vi "Test Dataset.vi"(11 "Enum":T1(ring)) -> (0 "error out":errorcluster, 2 "Parameters out":dbl[](array[numeric])=[-9.0, -8.75, -8.5, -8.25, -8.0, -7.75, -7.5, -7.25, -7.0, -6.75, -6.5, -6.25, -6.0, -5.75, -5.5, -5.25, -5.0, -4.75, -4.5, -4.25, -4.0, -3.75, -3.5, -3.25, -3.0, -2.75, -2.5, -2.25, -2.0, -1.75, -1.5, -1.25, -1.0, -0.75, -0.5, -0.25, 0.0, 0.25, 0.5, 0.75, 1.0, 1.25, 1.5, 1.75, 2.0, 2.25, 2.5, 2.75, 3.0, 3.25, 3.5, 3.75, 4.0, 4.25, 4.5, 4.75, 5.0, 5.25, 5.5, 5.75, 6.0, 6.25, 6.5, 6.75, 7.0, 7.25, 7.5, 7.75, 8.0, 8.25, 8.5, 8.75, 9.0], 3 "XY-data out":cluster{"X-array":dbl[], "Y-array":dbl[]}[](array[cluster]) {"Y-array" format="%.2p"; "X-array" format="%.2p"})   [LabVIEW 2019, in "xy_utilities.lvlib"]
uses:
  <vilib>/Utility/miscctls.llb/LVOffsetAndMultiplierTypeDef.ctl
  subVIs/Append (multiple).vi
  subVIs/Subtract float (multiple).vi
  subVIs/Append (single).vi
  subVIs/Append (double array).vi
  xy_utilities.lvlib
panel:
  out "XY graph":cluster{"Wavenumber":dbl[], "Data":dbl[]}[](graph)
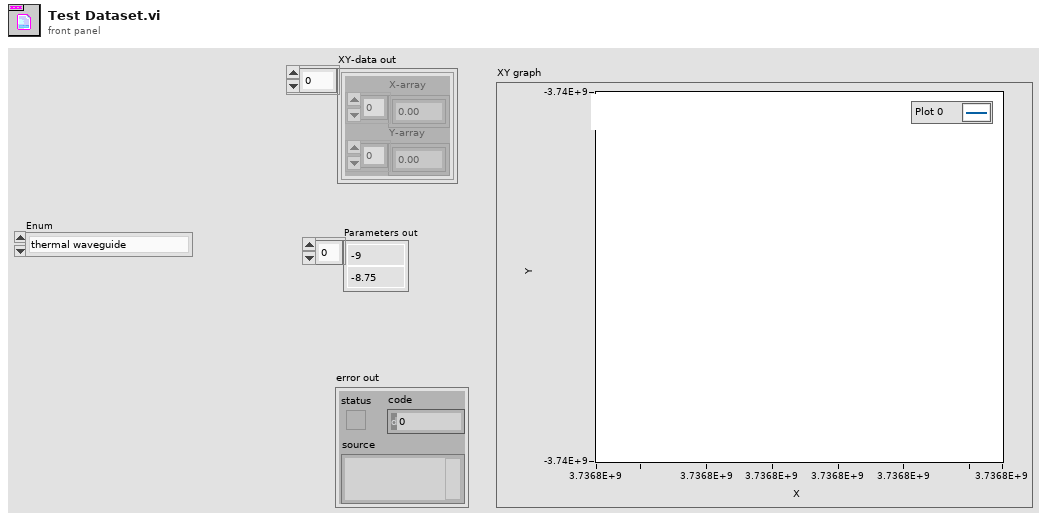
[diagram p1: front panel]
types:
  T1 = enum16{"thermal waveguide", "superlattice waveguide", "decay in atmosphere"}
  T2 = typedef "LVOffsetAndMultiplierTypeDef.ctl" = cluster{"Offset":dbl, "Multiplier":dbl}
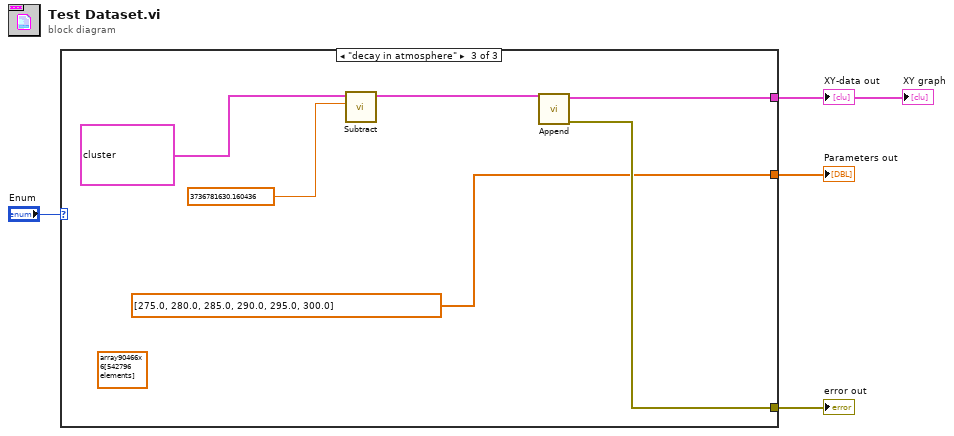
[diagram p0: block diagram]
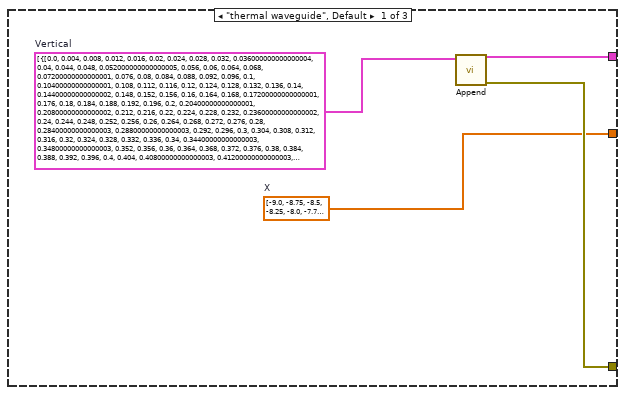
[diagram p2: hidden frame]
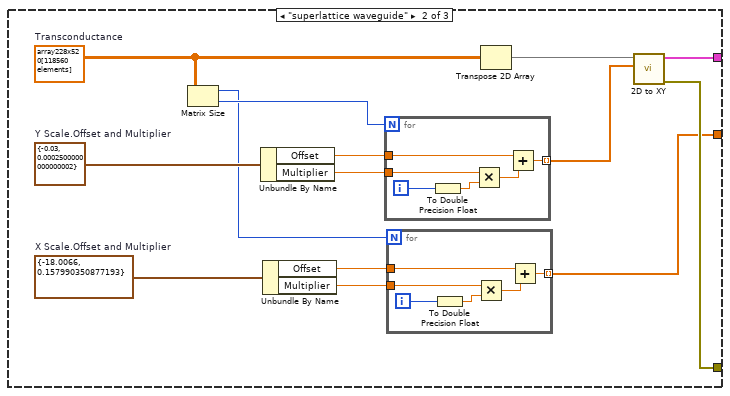
[diagram p3: hidden frame]
diagram:
  n1 = case shown="\"decay in atmosphere\"" "Enum" {
    tunnel: [w8 w10 w39] -> w4
    tunnel: [w7 w9 dbl[] [275.0, 280.0, 285.0, 290.0, 295.0, 300.0] ("X")] -> w3
    tunnel: [w5 w11 w40] -> w1
    frame "thermal waveguide", Default {
      w7 = dbl[] [-9.0, -8.75, -8.5, -8.25, -8.0, -7.75, -7.5, -7.25, -7.0, -6.75, -6.5, -6.25, -6.0, -5.75, -5.5, -5.25, -5.0, -4.75, -4.5, -4.25, -4.0, -3.75, -3.5, -3.25, -3.0, -2.75, -2.5, -2.25, -2.0, -1.75, -1.5, -1.25, -1.0, -0.75, -0.5, -0.25, 0.0, 0.25, 0.5, 0.75, 1.0, 1.25, 1.5, 1.75, 2.0, 2.25, 2.5, 2.75, 3.0, 3.25, 3.5, 3.75, 4.0, 4.25, 4.5, 4.75, 5.0, 5.25, 5.5, 5.75, 6.0, 6.25, 6.5, 6.75, 7.0, 7.25, 7.5, 7.75, 8.0, 8.25, 8.5, 8.75, 9.0]  # X
      w6 = cluster{"Intensity Data":dbl[], "Array":dbl[]}[] [{"Intensity Data"=[0.0, 0.004, 0.008, 0.012, 0.016, 0.02, 0.024, 0.028, 0.032, 0.036000000000000004, 0.04, 0.044, 0.048, 0.052000000000000005, 0.056, 0.06, 0.064, 0.068, 0.07200000000000001, 0.076, 0.08, 0.084, 0.088, 0.092, 0.096, 0.1, 0.10400000000000001, 0.108, 0.112, 0.116, 0.12, 0.124, 0.128, 0.132, 0.136, 0.14, 0.14400000000000002, 0.148, 0.152, 0.156, 0.16, 0.164, 0.168, 0.17200000000000001, 0.176, 0.18, 0.184, 0.188, 0.192, 0.196, 0.2, 0.20400000000000001, 0.20800000000000002, 0.212, 0.216, 0.22, 0.224, 0.228, 0.232, 0.23600000000000002, 0.24, 0.244, 0.248, 0.252, 0.256, 0.26, 0.264, 0.268, 0.272, 0.276, 0.28, 0.28400000000000003, 0.28800000000000003, 0.292, 0.296, 0.3, 0.304, 0.308, 0.312, 0.316, 0.32, 0.324, 0.328, 0.332, 0.336, 0.34, 0.34400000000000003, 0.34800000000000003, 0.352, 0.356, 0.36, 0.364, 0.368, 0.372, 0.376, 0.38, 0.384, 0.388, 0.392, 0.396, 0.4, 0.404, 0.40800000000000003, 0.41200000000000003, 0.41600000000000004, 0.42, 0.424, 0.428, 0.432, 0.436, 0.44, 0.444, 0.448, 0.452, 0.456, 0.46, 0.464, 0.468, 0.47200000000000003, 0.47600000000000003, 0.48, 0.484, 0.488, 0.492, 0.496, 0.5, 0.504, 0.508, 0.512, 0.516, 0.52, 0.524, 0.528, 0.532, 0.536, 0.54, 0.544, 0.548, 0.552, 0.556, 0.56, 0.5640000000000001, 0.5680000000000001, 0.5720000000000001, 0.5760000000000001, 0.58, 0.584, 0.588, 0.592, 0.596, 0.6, 0.604, 0.608, 0.612, 0.616, 0.62, 0.624, 0.628, 0.632, 0.636, 0.64, 0.644, 0.648, 0.652, 0.656, 0.66, 0.664, 0.668, 0.672, 0.676, 0.68, 0.684, 0.6880000000000001, 0.6920000000000001, 0.6960000000000001, 0.7000000000000001, 0.704, 0.708, 0.712, 0.716, 0.72, 0.724, 0.728, 0.732, 0.736, 0.74, 0.744, 0.748, 0.752, 0.756, 0.76, 0.764, 0.768, 0.772, 0.776, 0.78, 0.784, 0.788, 0.792, 0.796, 0.8, 0.804, 0.808, 0.812, 0.8160000000000001, 0.8200000000000001, 0.8240000000000001, 0.8280000000000001, 0.8320000000000001, 0.836, 0.84, 0.844, 0.848, 0.852, 0.856, 0.86, 0.864, 0.868, 0.872, 0.876, 0.88], "Array"=[1.68063e-07, 1.37198e-07, 8.79687e-08, 1.06463e-07, 1.07999e-07, 1.50443e-07, 1.6136e-07, 1.60216e-07, 1.51628e-07, 1.62347e-07, 2.24052e-07, 2.12498e-07, 1.69888e-07, 2.07771e-07, 2.10504e-07, 1.16164e-07, 1.03648e-07, 1.88353e-07, 2.52956e-07, 1.81322e-07, 1.3598e-07, 1.93502e-07, 3.06623e-07, 1.81397e-07, 1.56136e-07, 7.65771e-08, 1.0323e-07, 2.25052e-07, 2.18994e-07, 1.48687e-07, 1.23465e-07, 1.94812e-07, 8.89733e-08, 1.01215e-07, 1.91375e-07, 1.83998e-07, 1.70281e-07, 2.66741e-07, 1.84557e-07, 1.35922e-07, 1.53284e-07, 1.28241e-07, 1.84801e-07, 1.04068e-07, 8.03285e-08, 1.04402e-07, 8.12206e-08, 5.15301e-08, 2.02427e-07, 1.78907e-07, 1.0348e-07, 8.96397e-08, 1.49064e-07, 2.10614e-07, 1.94321e-07, 1.23458e-07, 2.49381e-08, 1.85551e-07, 1.98644e-07, 2.30779e-07, 3.77495e-07, 6.72036e-07, 1.17947e-06, 1.75588e-06, 2.53801e-06, 3.50995e-06, 4.10398e-06, 4.4421e-06, 4.54957e-06, 4.46684e-06, 4.29614e-06, 4.03689e-06, 3.7785e-06, 3.52652e-06, 3.3015e-06, 3.0176e-06, 2.73351e-06, 2.48081e-06, 2.28944e-06, 2.06704e-06, 1.80961e-06, 1.62787e-06, 1.44499e-06, 1.27341e-06, 1.12003e-06, 1.00442e-06, 8.63595e-07, 7.29893e-07, 6.0347e-07, 5.41881e-07, 4.90755e-07, 4.14075e-07, 3.64346e-07, 3.41478e-07, 3.11551e-07, 2.93279e-07, 3.09014e-07, 3.23829e-07, 3.14767e-07, 3.13298e-07, 3.2943e-07, 3.73559e-07, 3.85052e-07, 4.12776e-07, 4.52513e-07, 4.63779e-07, 5.00565e-07, 5.25226e-07, 5.28226e-07, 5.09122e-07, 4.69838e-07, 4.77525e-07, 4.87608e-07, 4.64681e-07, 4.29366e-07, 4.10075e-07, 3.911e-07, 3.53091e-07, 3.11529e-07, 2.80052e-07, 2.48962e-07, 2.2069e-07, 2.00389e-07, 1.80056e-07, 1.71025e-07, 1.52747e-07, 1.20455e-07, 1.10317e-07, 1.22804e-07, 1.19285e-07, 1.05556e-07, 1.00514e-07, 1.16004e-07, 1.33715e-07, 1.48638e-07, 1.67858e-07, 1.60768e-07, 1.72191e-07, 1.90163e-07, 2.12957e-07, 2.27031e-07, 2.42395e-07, 2.5957e-07, 2.75457e-07, 2.81378e-07, 2.87991e-07, 2.8598e-07, 2.99029e-07, 3.10983e-07, 2.98582e-07, 2.92597e-07, 2.96466e-07, 2.75316e-07, 2.60924e-07, 2.73094e-07, 2.76228e-07, 2.69051e-07, 2.49348e-07, 2.40239e-07, 2.38694e-07, 2.46997e-07, 2.3754e-07, 2.31936e-07, 2.37921e-07, 2.4129e-07, 2.36577e-07, 2.27175e-07, 2.23179e-07, 2.32753e-07, 2.22017e-07, 2.21659e-07, 2.35338e-07, 2.45551e-07, 2.48375e-07, 2.61624e-07, 2.68417e-07, 2.63606e-07, 2.83272e-07, 2.96328e-07, 2.89196e-07, 2.96568e-07, 3.03707e-07, 3.06523e-07, 3.1915e-07, 3.12655e-07, 2.95357e-07, 2.95008e-07, 2.98448e-07, 3.09012e-07, 3.01923e-07, 2.96206e-07, 3.10244e-07, 3.04155e-07, 2.92192e-07, 2.85057e-07, 2.82269e-07, 2.90168e-07, 2.75276e-07, 2.42554e-07, 2.36848e-07, 2.39448e-07, 2.14838e-07, 2.06682e-07, 2.0462e-07, 1.85893e-07, 1.77192e-07, 1.71389e-07, 1.56772e-07, 1.51419e-07, 1.47796e-07, 1.53989e-07, 1.38128e-07, 1.40478e-07, 1.52301e-07, 1.42379e-07, 1.31716e-07, 1.3604e-07, 1.51662e-07, 1.43388e-07, 1.35586e-07, 1.45146e-07]}, ...(73 in all)]  # Vertical
      n2 = call-poly "Append.vi"("XY-data (A)"=w6) -> ("error out"=w8:errorcluster, "XY-data out"=w5:cluster{"X-array":dbl[], "Y-array":dbl[]}[])  [unwired: 9 in]
    }
    frame "superlattice waveguide" {
      w16 = T2 {"Offset"=-0.03, "Multiplier"=0.0002500000000000002}  # Y Scale.Offset and Multiplier
      w19 = T2 {"Offset"=-18.0066, "Multiplier"=0.157990350877193}  # X Scale.Offset and Multiplier
      w20 = dbl[][] array228x520[118560 elements]  # Transconductance
      n3 = Matrix Size(0:w20) -> (1:w14:i32, 2:w15:i32)
      n4 = Unbundle By Name(w16) -> ("Offset"=w18:dbl, "Multiplier"=w17:dbl)
      n5 = Unbundle By Name(w19) -> ("Offset"=w21:dbl, "Multiplier"=w22:dbl)
      n6 = for {
        N: w15 -> [_]
        tunnel: w18 -> [w26]
        tunnel: w17 -> [w28]
        tunnel: [w25] -> w12 mode=indexing
        i -> [w27]
        n7 = To Double Precision Float(number=w27) -> (double precision float=w24:dbl)
        n8 = Multiply(x=w28, y=w24) -> (x*y=w23:dbl)
        n9 = Add(x=w26, y=w23) -> (x+y=w25:dbl)
      }
      n10 = for {
        N: w14 -> [_]
        tunnel: w21 -> [w32]
        tunnel: w22 -> [w34]
        tunnel: [w31] -> w9 mode=indexing
        i -> [w33]
        n11 = To Double Precision Float(number=w33) -> (double precision float=w30:dbl)
        n12 = Multiply(x=w34, y=w30) -> (x*y=w29:dbl)
        n13 = Add(x=w32, y=w29) -> (x+y=w31:dbl)
      }
      n14 = Transpose 2D Array(2D array=w20) -> (transposed array=w13:dbl[][])
      n15 = call "2D to XY.vi"("X Array"=w12, "2D Z Array"=w13) -> ("error out"=w10:errorcluster, "XY-data out"=w11:cluster{"X-array":dbl[], "Y-array":dbl[]}[])  [unwired: 8 in]
    }
    frame "decay in atmosphere" {
      (unwired) dbl[][] array90466x6[542796 elements] ("Data Intensity")
      n16 = call-poly "Subtract.vi"("x (0)"=3736781630.160436 ("y"), "XY-data"=cluster{"Intensity Data":dbl[], "Array":dbl[]}[] [{"Intensity Data"=array[14499 elements], "Array"=array[14499 elements]}, {"Intensity Data"=array[14553 elements], "Array"=array[14553 elements]}, {"Intensity Data"=array[14670 elements], "Array"=array[14670 elements]}, {"Intensity Data"=array[14716 elements], "Array"=array[14716 elements]}, {"Intensity Data"=array[14637 elements], "Array"=array[14637 elements]}, {"Intensity Data"=array[14706 elements], "Array"=array[14706 elements]}] ("XY Graph: Unprocessed")) -> ("XY-data out"=w36:cluster{"X-array":dbl[], "Y-array":dbl[]}[])  [unwired: 8 in, 1 out]
      n17 = call-poly "Append.vi"("XY-data (A)"=w36) -> ("error out"=w39:errorcluster, "XY-data out"=w40:cluster{"X-array":dbl[], "Y-array":dbl[]}[])  [unwired: 9 in]
    }
  }
  "XY-data out" <- w1
  "error out" <- w4
  "Parameters out" <- w3
  "XY graph" <- w1
